vi "Write DMA.vi"(8 "error in (no error)":errorcluster, 10 "DMA Ref":T1, 11 "Waveform Refs":refnum<class "Single Waveform Read (DBL).lvclass">[](array[class])) -> (0 "error out":errorcluster, 1 "Empty Elements Remaining":u32, 2 "DMA Ref":T1, 3 "Waveform Refs":refnum<class "Single Waveform Read (DBL).lvclass">[](array[class]))   [LabVIEW 2016, in "FPGA Addon Engine.lvlib"]
uses:
  FPGA Addon Engine.lvlib
  Types/DMA Output Ref.ctl
  <vilib>/NI Veristand/Custom Device Waveform API/Single Waveform Read (DBL)/Single Waveform Read (DBL).lvclass
  C:/Program Files (x86)/National Instruments/LabVIEW 2016/vi.lib/NI Veristand/Custom Device Waveform API/Waveform Session.lvclass
  <vilib>/NI Veristand/Custom Device Waveform API/Waveform Session.lvclass/Waveform Session.ctl
  <vilib>/NI Veristand/Custom Device Waveform API/Single Waveform Read (DBL)/Single Waveform Read (DBL).lvclass/Single Waveform Read (DBL).ctl
  <vilib>/NI Veristand/Custom Device Waveform API/Internal Comm Classes/WPL Comm/WPL Comm (1D DBL)/WPL Comm (1D DBL).lvclass/WPL Comm (1D DBL).ctl
  <vilib>/NI Veristand/Custom Device Waveform API/Single Waveform Read (DBL)/NI VeriStand - Read Single Waveform (DBL).vi
  <vilib>/NI Veristand/Custom Device Waveform API/Internal Comm Classes/WPL Comm/WPL Comm (1D DBL)/Comm_read 1d dbl.vi
  <vilib>/NI Veristand/Custom Device Waveform API/Check Opened.vi
  <vilib>/NI Veristand/Custom Device Waveform API/Internal Comm Classes/WPL Comm/Convert Q Error to Shutdown Error.vi
  <vilib>/rvi/errors/niLvFpgaAdjustHostInterfaceError.vi
  <vilib>/Utility/error.llb/Error Cluster From Error Code.vi
  <vilib>/rvi/interface/nirviMethod/nirviMethod.xnode
  <vilib>/NI VeriStand/Custom Device Waveform API/NI_VS Custom Device Waveform API.lvlib
  <vilib>/FPGAPlugInAG/Dynamic/niLvFpga_WriteFifo_Dynamic.vi
  <vilib>/rvi/errors/niLvFpgaMergeErrorWithErrorCode.vi
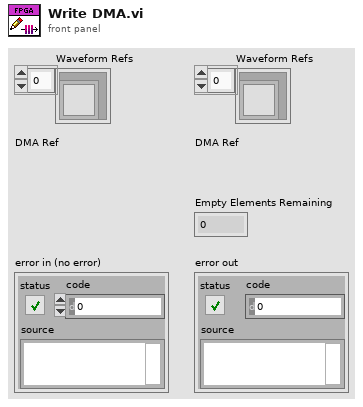
[diagram p1: front panel]
types:
  T1 = typedef "FPGA Addon Engine.lvlib/DMA Output Ref.ctl" = refnum<k20>
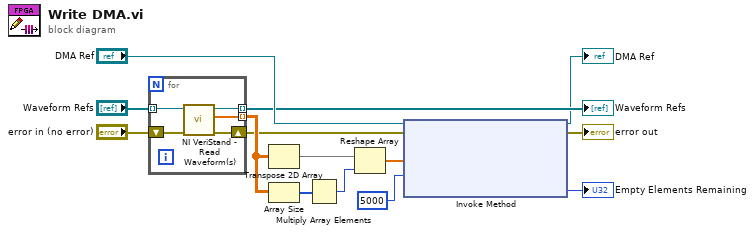
[diagram p0: block diagram]
diagram:
  n1 = for {
    tunnel: [w19] -> w3 mode=indexing
    shift-right: [w18] -> w2
    shift-left: "error in (no error)" -> [w17]
    tunnel: "Waveform Refs" -> [w16] mode=indexing
    tunnel: [w15] -> w8 mode=indexing
    n2 = call-poly <vilib>:"NI VeriStand - Read Waveform(s).vi"("error in (no error)"=w17, "Single Waveform Read Session (DBL) in"=w16) -> ("error out"=w18:errorcluster, "Data"=w19:dbl[], "Single Waveform Read Session (DBL) out"=w15:refnum<class "Single Waveform Read (DBL).lvclass">)  [unwired: 5 in, 2 out]
  }
  "Waveform Refs" <- w8
  n3 = Transpose 2D Array(2D array=w3) -> (transposed array=w4:dbl[][])
  n4 = Array Size(array=w3) -> (size(s)=w6:i32[])
  n5 = Multiply Array Elements(1:w6) -> (0:w5:i32)
  n6 = Reshape Array(w4, w5) -> (w11:dbl[])
  n7 = xnode "Invoke Method"("FPGA VI Reference In"="DMA Ref", "error in"=w2, "Data"=w11, "Timeout (ms)"=5000) -> ("FPGA VI Reference Out"=→"DMA Ref":T1, "error out"=→"error out":errorcluster, "Empty Elements Remaining"=→"Empty Elements Remaining":u32)
